vi "GenericStatusIndicator.vi"(9 "Total":i32, 10 "Current Iteration":i32, 11 "Status Indicator Ref In":refnum<vi>) -> (3 "CLI Status to Print":string)   [LabVIEW 2019, in "DepsWatch.lvlib"]
uses:
  DepsWatch.lvlib
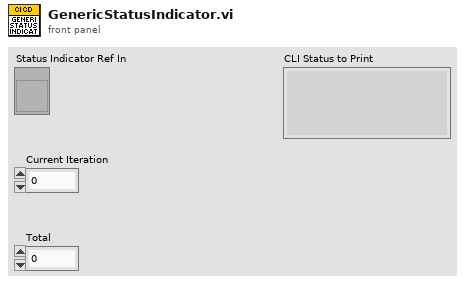
[diagram p1: front panel]
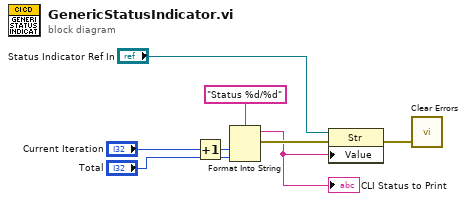
[diagram p0: block diagram]
diagram:
  n1 = Increment(x="Current Iteration") -> (x+1=w5:i32)
  n2 = Format Into String(format string="Status %d/%d", w5, "Total") -> (resulting string=w2:string, error out=w3:errorcluster)  [unwired: 2 in]
  "CLI Status to Print" <- w2
  n3 = property class="Str"(reference="Status Indicator Ref In", error in=w3, "Value"=w2) -> (error out=w1:errorcluster)  [unwired: 1 out]
  n4 = call <vilib>:"Clear Errors.vi"("error in (no error)"=w1) -> ()  [unwired: 5 in, 2 out]
